vi "Write MLVClient.vi"(8 "error in (no error)":errorcluster, 10 "MLVClient":refnum<k24>, 11 "MongoDB-Client in":refnum<class "MongoDB-Client.lvclass">) -> (0 "error out":errorcluster, 3 "MongoDB-Client out":refnum<class "MongoDB-Client.lvclass">)   [LabVIEW 2016, in "MongoDB-Client.lvlib" / "MongoDB-Client.lvclass"]
uses:
  MongoDB-Client.lvclass
  D:/Users/blume/Desktop/LV/MongoDB-Driver/MLV DLLs/MongoLabVIEW.dll
  LV/MongoDB-Driver/MLV DLLs/MongoLabVIEW.dll
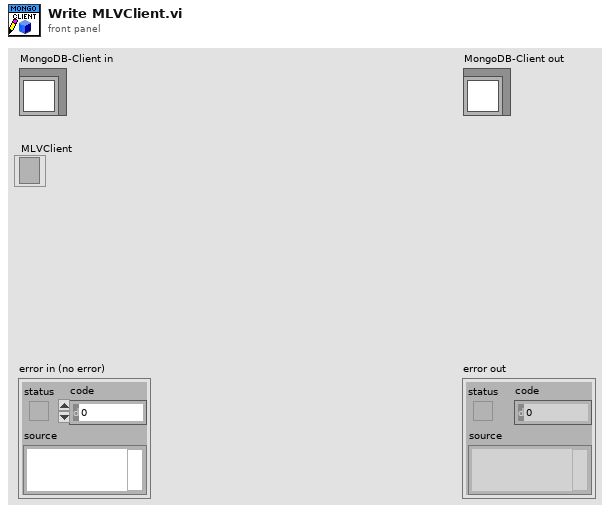
[diagram p1: front panel]
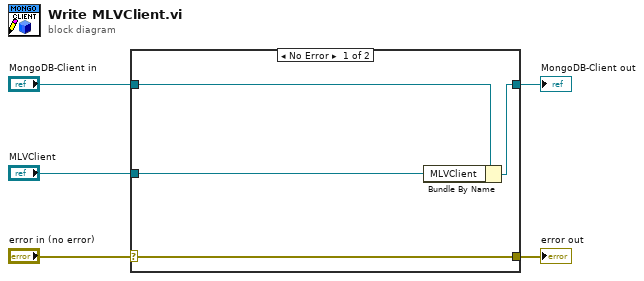
[diagram p0: block diagram]
diagram:
  n1 = case shown="No Error" "error in (no error)" {
    selector: "error in (no error)" -> [w9 w10]
    tunnel: [w9 w10] -> w4
    tunnel: [w7 w11] -> w2
    tunnel: "MongoDB-Client in" -> [w8 w11]
    tunnel: "MLVClient" -> [w6 _]
    frame No Error {
      n2 = Bundle By Name(cluster=w8, "MLVClient"=w6) -> (w7:refnum<class "MongoDB-Client.lvclass">)
    }
    frame Error {
    }
  }
  "error out" <- w4
  "MongoDB-Client out" <- w2
